vi "DCS_loc_at_point.vi"(0 "DCS 1 Loc":dbl[](array[numeric]), 1 "Distance from DCS 1":dbl, 2 "DCS 2 Loc":dbl[](array[numeric]), 3 "DCS 1 Corrections":dbl[](array[numeric])=[0.551, 0.25], 4 "DCS 2 Correections":dbl[](array[numeric])=[-2.152, -0.25]) -> (5 "Current Loc":dbl[](array[numeric]))   [LabVIEW 2015]
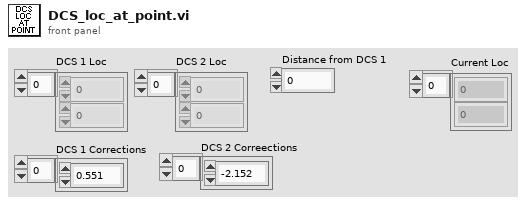
[diagram p1: front panel]
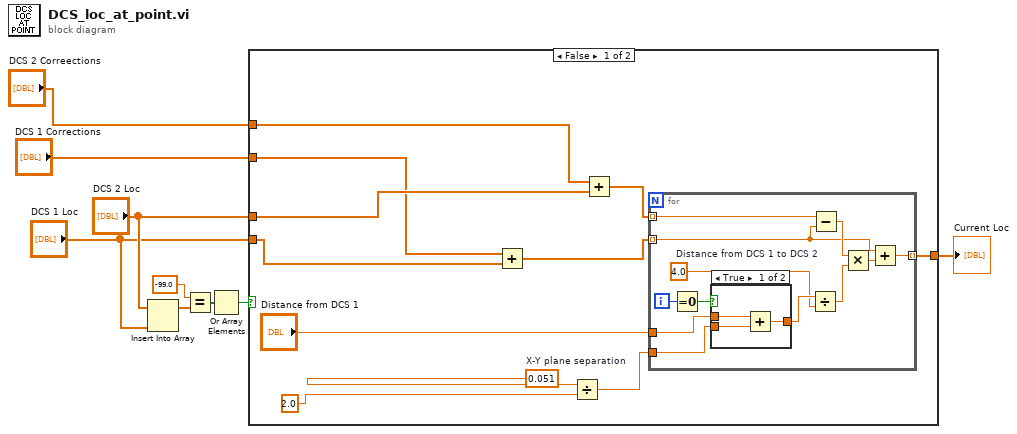
[diagram p0: block diagram]
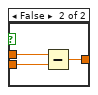
[diagram p2: hidden frame]
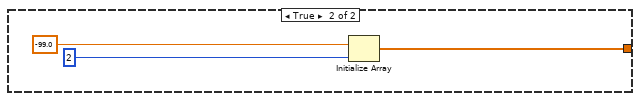
[diagram p3: hidden frame]
diagram:
  n1 = Insert Into Array(array="DCS 2 Loc", new element="DCS 1 Loc") -> (w5:dbl[])  [unwired: 1 in]
  n2 = Equal?(x=-99.0 ("y"), y=w5) -> (x = y?=w6:bool[])
  n3 = Or Array Elements(Boolean array=w6) -> (logical OR=w3:bool)
  n4 = case shown="False" w3 {
    tunnel: [w20 w39] -> w9
    tunnel: "DCS 1 Loc" -> [w15 _]
    tunnel: "DCS 2 Loc" -> [w13 _]
    tunnel: "DCS 2 Correections" -> [w11 _]
    tunnel: "DCS 1 Corrections" -> [w10 _]
    frame False {
      w19 = 0.051  # X-Y plane separation
      n5 = Add(x=w10, y=w15) -> (x+y=w14:dbl[])
      n6 = Divide(x=w19, y=2.0) -> (x/y=w16:dbl)
      n7 = Add(x=w11, y=w13) -> (x+y=w12:dbl[])
      n8 = for {
        tunnel: [w23] -> w20 mode=indexing
        tunnel: "Distance from DCS 1" -> [w31]
        tunnel: w16 -> [w30]
        tunnel: w14 -> [w22] mode=indexing
        tunnel: w12 -> [w29] mode=indexing
        i -> [w21]
        w27 = 4.0  # Distance from DCS 1 to DCS 2
        n9 = Equal To 0?(x=w21) -> (x = 0?=w32:bool)
        n10 = case shown="True" w32 {
          tunnel: w31 -> [w35 w38]
          tunnel: w30 -> [w34 w37]
          tunnel: [w33 w36] -> w28
          frame True {
            n11 = Add(x=w35, y=w34) -> (x+y=w33:dbl)
          }
          frame False {
            n12 = Subtract(x=w38, y=w37) -> (x-y=w36:dbl)
          }
        }
        n13 = Divide(x=w28, y=w27) -> (x/y=w26:dbl)
        n14 = Subtract(x=w29, y=w22) -> (x-y=w25:dbl)
        n15 = Multiply(x=w25, y=w26) -> (x*y=w24:dbl)
        n16 = Add(x=w22, y=w24) -> (x+y=w23:dbl)
      }
    }
    frame True {
      n17 = Initialize Array(-99.0 ("y"), 2 ("dimension size")) -> (w39:dbl[])
    }
  }
  "Current Loc" <- w9
